vi "Standard Joystick Control.vi"() -> ()   [LabVIEW 2016, in "Aerotech VIs.lvlib"]
uses:
  Aerotech VIs.lvlib
  Motion/EnableMultiple.vi
  Motion/HomeSingle.vi
  Motion/MoveAbsMultiple.vi
  Motion/FaultAckMultiple.vi
  Motion/DisableMultiple.vi
panel:
  in  "PC Board Position":bool
  in  "Plate Position":bool
  in  "Silicon Position":bool
  out "Vacuum Working":bool[](array[boolean])
  in  "Vacuum On/Off":bool[](array[boolean])
  out "z vel units":string
  out "y vel units":string
  out "x vel units":string
  out "u vel units":string
  out "Z - Velocity":dbl
  out "Y - Velocity":dbl
  out "X - Velocity":dbl
  out "U - Velocity":dbl
  in  "Fault Acknowledged":bool
  in  "joystick reset":bool
  in  "joystick on":bool
  in  "stop":bool
  in  "z home":bool
  in  "y home":bool
  in  "x home":bool
  in  "u home":bool
  out "units 4":string
  out "units 3":string
  out "units 2":string
  out "units":string
  out "Z - Position":dbl
  out "Y - Position":dbl
  out "X - Position":dbl
  out "U - Position":dbl
  out "Z - Axis Status":string
  out "Y - Axis Status":string
  out "X - Axis Status":string
  out "U - Axis Status":string
  # "If vacuum sensor\nshows a green\nlight when turned\noffthen it means it\nis not wired correctly"
  # "Vacuum Controls"
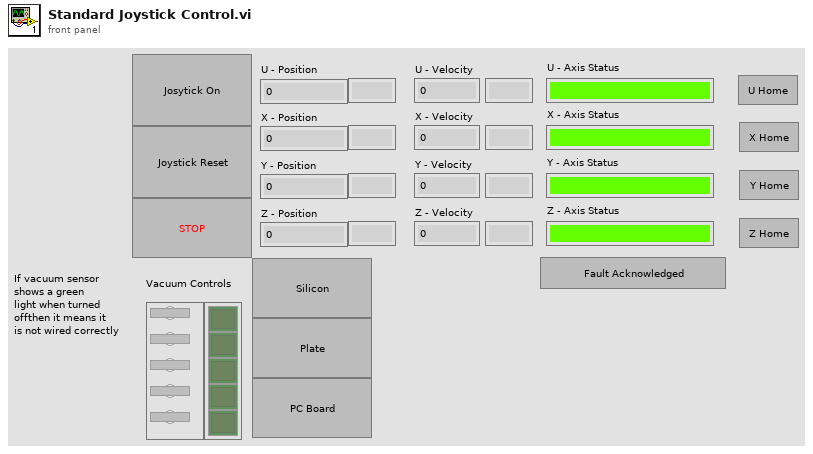
[diagram p1: front panel]
types:
  T1 = typedef "AxisDiagPacket.ctl" = cluster{"Axis Name":string, "Analog Input 0":dbl, "Analog Input 1":dbl, "Axis Fault (num)":i32, "Axis Fault (str)":string, "Axis Fault (bits)":cluster{"AmplifierFault":bool, "AmplifierTemperatureFault":bool, "CcwEndOfTravelLimitFault":bool, "CcwSoftwareLimitFault":bool, "CommunicationLostFault":bool, "CwEndOfTravelLimitFault":bool, "CwSoftwareLimitFault":bool, "EmergencyStopFault":bool, "EncoderFault":bool, "ExternalFault":bool, "FeedbackScalingFault":bool, "GantryMisalignFault ":bool, "HallSensorFault":bool, "InPositionTimeoutFault":bool, "MarkerSearchFault":bool, "MaxVelocityCommandFault":bool, "MotorTemperatureFault":bool, "None":bool, "OverCurrentFault":bool, "PositionErrorFault":bool, "PositionFeedbackFault":bool, "ProbeInputFault":bool, "SafeZoneFault":bool, "VelocityErrorFault":bool, "VelocityFeedbackFault":bool, "VoltageClampFault":bool, "PowerSupplyFault":bool}, "Axis Status (num)":i32, "Axis Status (str)":string, "Axis Status (bits)":cluster{"BacklashActive":bool, "CalibrationEnabled1D":bool, "CalibrationEnabled2D":bool, "CommandValid":bool, "DriveAbortPending":bool, "DrivePending":bool, "Enabling":bool, "GainMappingEnabled":bool, "GantryAligned":bool, "GantryRealigning":bool, "Homed":bool, "Homing":bool, "IFOVEnabled":bool, "Jogging":bool, "JogGenerating":bool, "JoystickControl":bool, "MasterSlaveControl":bool, "MotionBlocked":bool, "MotionClamped":bool, "MoveDone":bool, "None":bool, "NotVirtual":bool, "Profiling":bool, "Stability0":bool, "Stability1":bool, "TrajectoryFiltering":bool, "WaitDone":bool}, "Current Command":sgl, "Current Error":sgl, "Current Feedback":sgl, "Digital Inputs":i32, "Digital Outputs":i32, "Drive Status":i32, "Drive Status (str)":string, "Drive Status (bits)":cluster{"AccelerationPhase":bool, "AutofocusActive":bool, "BrakeOutput":bool, "CcwEndOfTravelLimitInput":bool, "CosineEncoderError":bool, "CurrentClamp":bool, "CwEndOfTravelLimitInput":bool, "DecelerationPhase":bool, "DualLoopActive":bool, "EmergencyStopInput":bool, "Enabled":bool, "EncoderClipping":bool, "GalvoCalibrationEnabled":bool, "GalvoPowerCorrection":bool, "HallAInput":bool, "HallBInput":bool, "HallCInput":bool, "HighResolutionMode":bool, "HomeLimitInput":bool, "InPosition":bool, "InPosition2":bool, "MarkerInput":bool, "MarkerLatch":bool, "MoveActive":bool, "NoMotorSupply":bool, "None":bool, "PowerLimiting":bool, "ProgrammingFlash":bool, "ProgrammingMXH":bool, "PSOHaltLatch":bool, "ServoControl":bool, "SineEncoderError":bool}, "Position Feedback Auxiliary":dbl, "Position Command":dbl, "Position Error":dbl, "Position Feedback":dbl, "Program Position Command":dbl, "Program Position Error":dbl, "Program Position Feedback":dbl, "Velocity Command":dbl, "Velocity Error":dbl, "Velocity Feedback":dbl}
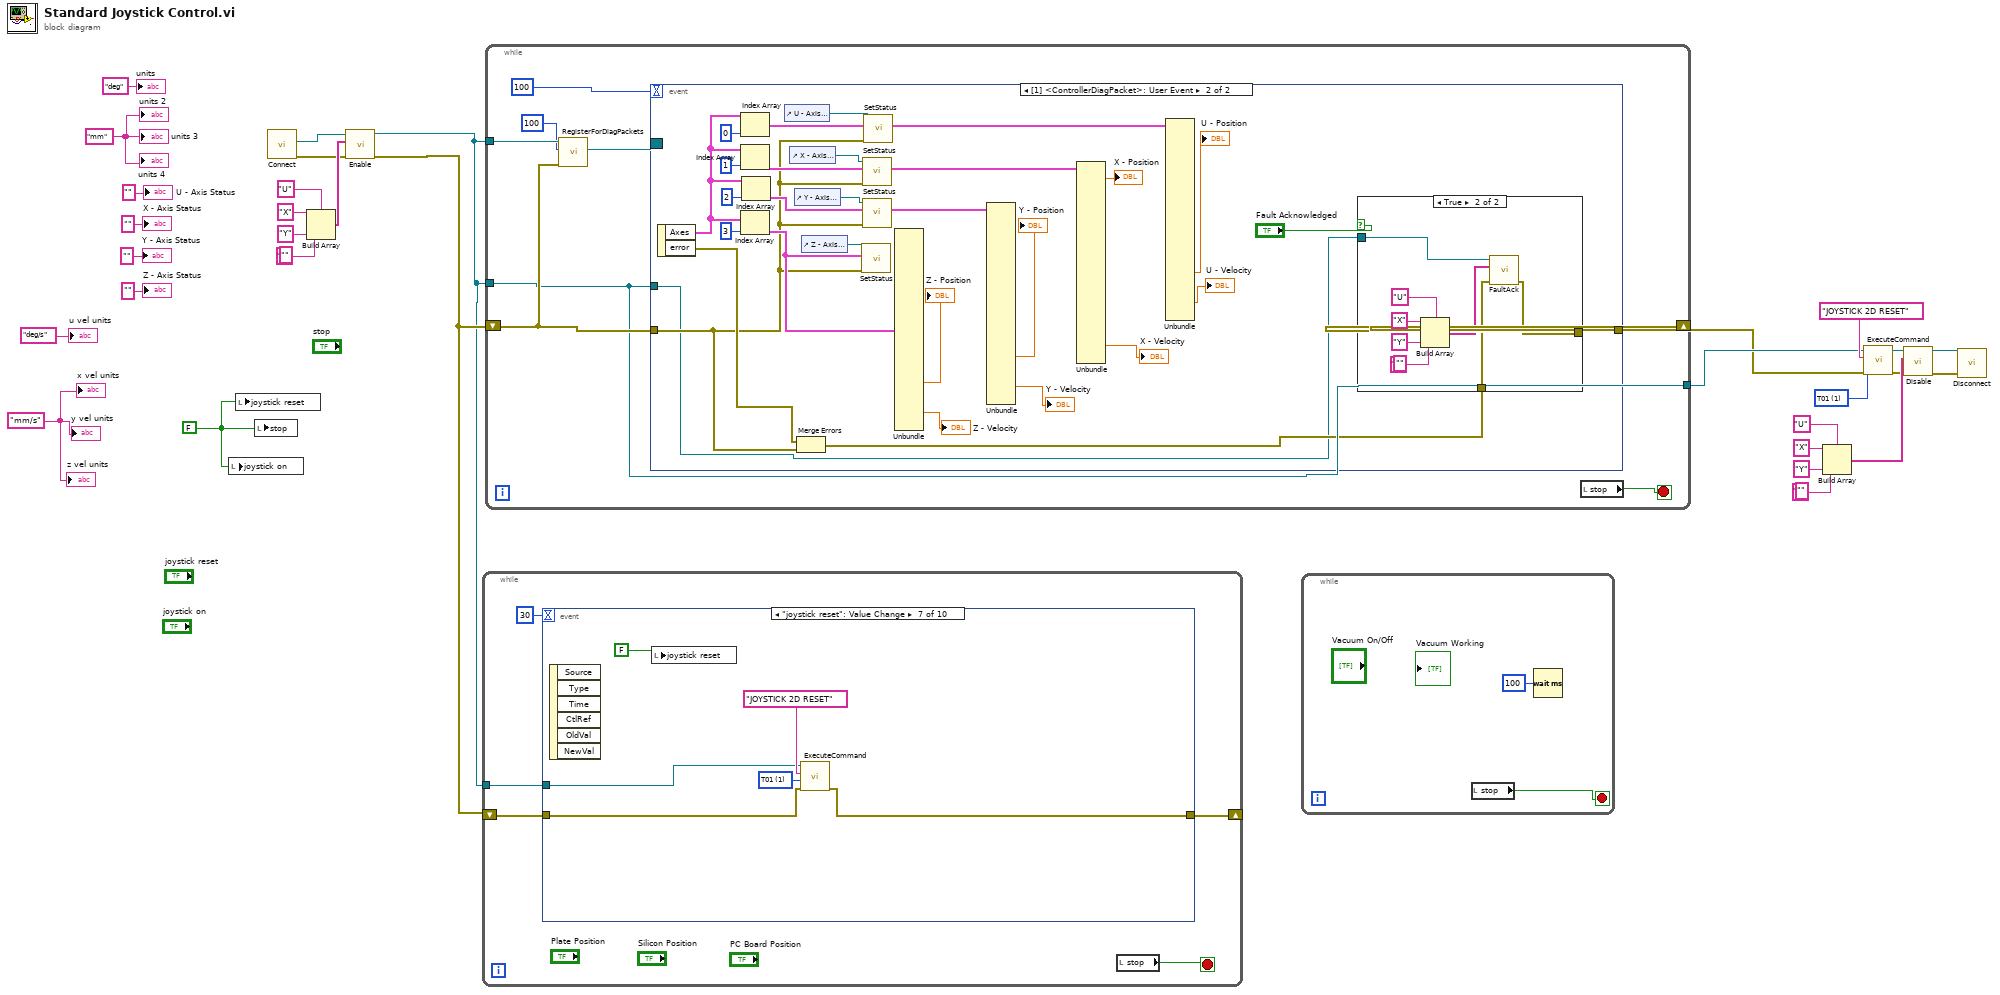
[diagram p0: block diagram]
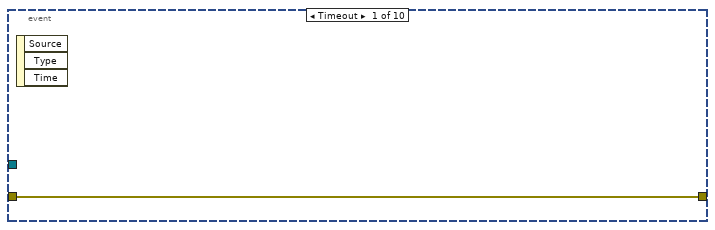
[diagram p2: hidden frame]
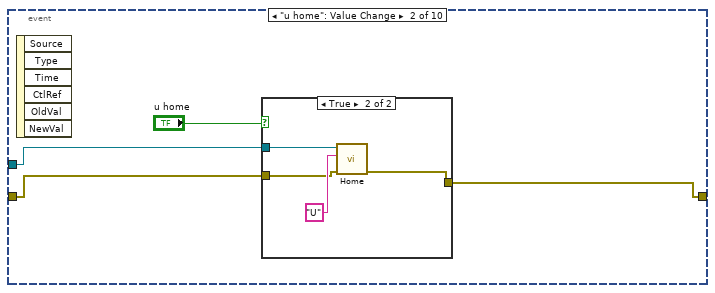
[diagram p3: hidden frame]
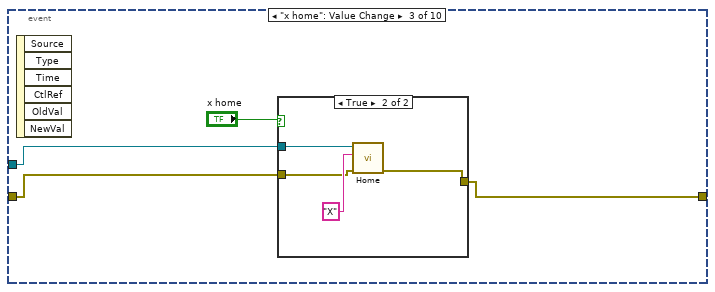
[diagram p5: hidden frame]
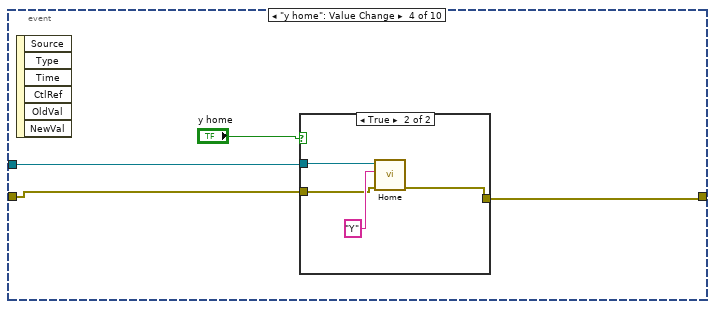
[diagram p7: hidden frame]
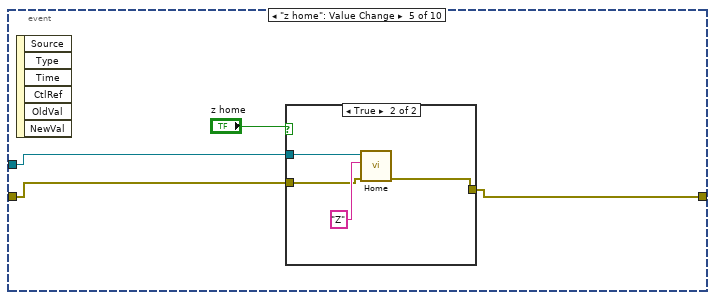
[diagram p9: hidden frame]
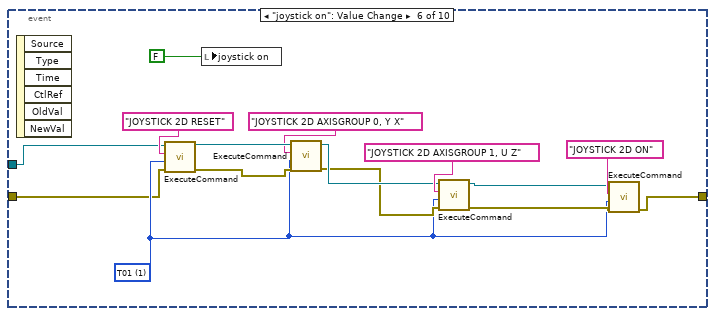
[diagram p11: hidden frame]
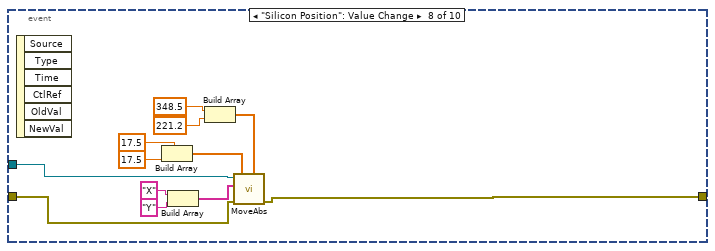
[diagram p12: hidden frame]
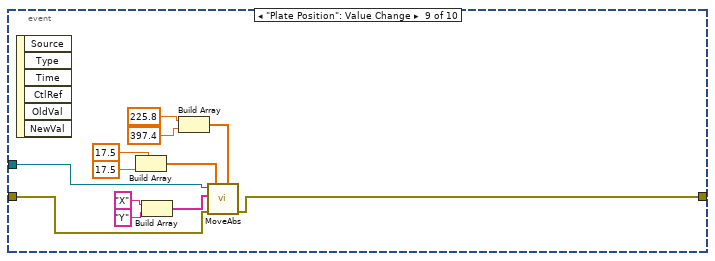
[diagram p13: hidden frame]
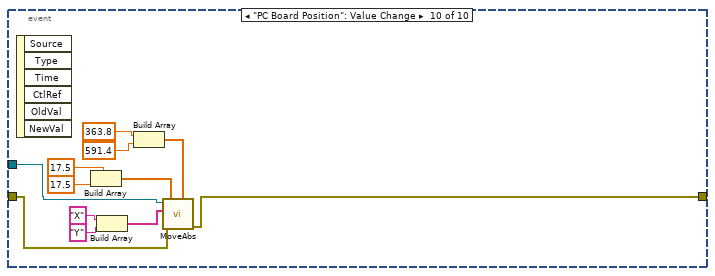
[diagram p14: hidden frame]
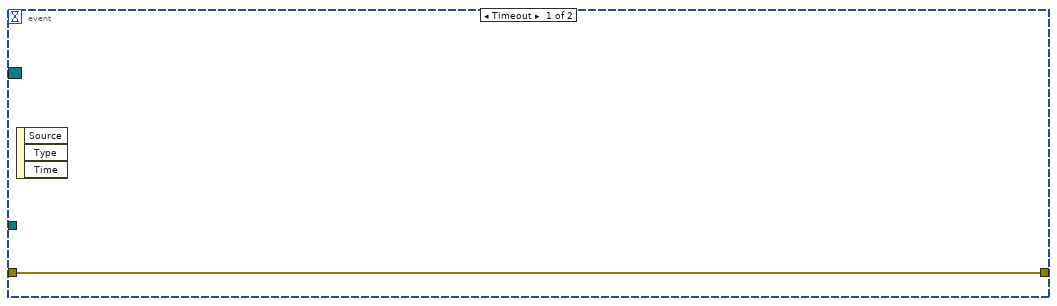
[diagram p15: hidden frame]
diagram:
  w9 = 1 items=["TLibrary", "T01", "T02", "T03", "T04", "T05", "T06", "T07", "T08", "T09", "T10", "T11", "T12", "T13", "T14", "T15", "T16", "T17", "T18", "T19", "T20", "T21", "T22", "T23", "T24", "T25", "T26", "T27", "T28", "T29", "T30", "T31"] ("taskId")
  w10 = "mm/s"
  w12 = FALSE
  (unwired) ""
  w19 = "mm"
  (unwired) ""
  n1 = local write "joystick on"(w12) -> ()
  n2 = local write "joystick reset"(w12) -> ()
  n3 = local write "stop"(w12) -> ()
  n4 = call "Connect.vi"() -> ("error out"=w22:errorcluster, "controller"=w21:refnum<k24>)  [unwired: 10 in]
  n5 = Build Array("U", "X", "Y", "Z") -> (w27:string[])
  n6 = call-poly "Enable.vi"("error in (no error)"=w22, "axis names"=w27, "controller in"=w21) -> ("error out"=w2:errorcluster, "controller out"=w1:refnum<k24>)  [unwired: 7 in]
  n7 = while {
    shift-right: [w35] -> _
    shift-left: w2 -> [w36]
    tunnel: w1 -> [w33]
    stop <- w32 stop-if-true
    n8 = event shown="[6] \"joystick reset\": Value Change" {
      selector: _ -> [_ _ _ _ _ _ _ _ _ _]
      dyn-events: _ -> [_ _ _ _ _ _ _ _ _ _]
      timeout: 30 -> [_ _ _ _ _ _ _ _ _ _]
      tunnel: w36 -> [w37 w41 w50 w59 w68 w75 w91 w105 w108 w120]
      tunnel: [w37 w40 w49 w58 w66 w74 w90 w104 w107 w119] -> w35
      tunnel: w33 -> [_ w39 w48 w57 w67 w76 w92 w106 w109 w121]
      event Timeout {
        n9 = event-data() -> ()  [unwired: 1 in, 3 out]
      }
      event "u home": Value Change {
        n10 = event-data() -> ()  [unwired: 1 in, 6 out]
        n11 = case shown="True" "u home" {
          tunnel: w41 -> [w42 w45]
          tunnel: [w42 w44] -> w40
          tunnel: w39 -> [_ w43]
          frame False {
          }
          frame True {
            n12 = call-poly "Home.vi"("error in (no error)"=w45, "axis name"="U", "controller in"=w43) -> ("error out"=w44:errorcluster)  [unwired: 7 in, 1 out]
          }
        }
      }
      event "x home": Value Change {
        n13 = event-data() -> ()  [unwired: 1 in, 6 out]
        n14 = case shown="True" "x home" {
          tunnel: w50 -> [w51 w54]
          tunnel: [w51 w53] -> w49
          tunnel: w48 -> [_ w52]
          frame False {
          }
          frame True {
            n15 = call-poly "Home.vi"("error in (no error)"=w54, "axis name"="X", "controller in"=w52) -> ("error out"=w53:errorcluster)  [unwired: 7 in, 1 out]
          }
        }
      }
      event "y home": Value Change {
        n16 = event-data() -> ()  [unwired: 1 in, 6 out]
        n17 = case shown="True" "y home" {
          tunnel: w59 -> [w60 w63]
          tunnel: [w60 w62] -> w58
          tunnel: w57 -> [_ w61]
          frame False {
          }
          frame True {
            n18 = call-poly "Home.vi"("error in (no error)"=w63, "axis name"="Y", "controller in"=w61) -> ("error out"=w62:errorcluster)  [unwired: 7 in, 1 out]
          }
        }
      }
      event "z home": Value Change {
        n19 = event-data() -> ()  [unwired: 1 in, 6 out]
        n20 = case shown="True" "z home" {
          tunnel: w68 -> [w69 w72]
          tunnel: [w69 w71] -> w66
          tunnel: w67 -> [_ w70]
          frame False {
          }
          frame True {
            n21 = call-poly "Home.vi"("error in (no error)"=w72, "axis name"="Z", "controller in"=w70) -> ("error out"=w71:errorcluster)  [unwired: 7 in, 1 out]
          }
        }
      }
      event "joystick on": Value Change {
        w77 = 1 items=["TLibrary", "T01", "T02", "T03", "T04", "T05", "T06", "T07", "T08", "T09", "T10", "T11", "T12", "T13", "T14", "T15", "T16", "T17", "T18", "T19", "T20", "T21", "T22", "T23", "T24", "T25", "T26", "T27", "T28", "T29", "T30", "T31"] ("taskId")
        n22 = event-data() -> ()  [unwired: 1 in, 6 out]
        n23 = call "ExecuteCommand.vi"("error in (no error)"=w75, "taskId"=w77, "Command Code"="JOYSTICK 2D RESET", "controller in"=w76) -> ("error out"=w86:errorcluster, "controller out"=w87:refnum<k24>)  [unwired: 5 in, 1 out]
        n24 = local write "joystick on"(FALSE) -> ()
        n25 = call "ExecuteCommand.vi"("error in (no error)"=w86, "taskId"=w77, "Command Code"="JOYSTICK 2D AXISGROUP 0, Y X", "controller in"=w87) -> ("error out"=w82:errorcluster, "controller out"=w83:refnum<k24>)  [unwired: 5 in, 1 out]
        n26 = call "ExecuteCommand.vi"("error in (no error)"=w82, "taskId"=w77, "Command Code"="JOYSTICK 2D AXISGROUP 1, U Z", "controller in"=w83) -> ("error out"=w80:errorcluster, "controller out"=w79:refnum<k24>)  [unwired: 5 in, 1 out]
        n27 = call "ExecuteCommand.vi"("error in (no error)"=w80, "taskId"=w77, "Command Code"="JOYSTICK 2D ON", "controller in"=w79) -> ("error out"=w74:errorcluster)  [unwired: 5 in, 2 out]
      }
      event "joystick reset": Value Change {
        w94 = 1 items=["TLibrary", "T01", "T02", "T03", "T04", "T05", "T06", "T07", "T08", "T09", "T10", "T11", "T12", "T13", "T14", "T15", "T16", "T17", "T18", "T19", "T20", "T21", "T22", "T23", "T24", "T25", "T26", "T27", "T28", "T29", "T30", "T31"] ("taskId")
        n28 = event-data() -> ()  [unwired: 1 in, 6 out]
        n29 = local write "joystick reset"(FALSE) -> ()
        n30 = call "ExecuteCommand.vi"("error in (no error)"=w91, "taskId"=w94, "Command Code"="JOYSTICK 2D RESET", "controller in"=w92) -> ("error out"=w90:errorcluster)  [unwired: 5 in, 2 out]
      }
      event "Silicon Position": Value Change {
        n31 = event-data() -> ()  [unwired: 1 in, 6 out]
        n32 = Build Array(17.5, 17.5) -> (w101:dbl[])
        n33 = Build Array("X", "Y") -> (w98:string[])
        n34 = Build Array(348.5, 221.2) -> (w95:dbl[])
        n35 = call-poly "MoveAbs.vi"("positions"=w95, "speeds"=w101, "error in (no error)"=w105, "axis names"=w98, "controller in"=w106) -> ("error out"=w104:errorcluster)  [unwired: 5 in, 1 out]
      }
      event "Plate Position": Value Change {
        n36 = event-data() -> ()  [unwired: 1 in, 6 out]
        n37 = Build Array(17.5, 17.5) -> (w116:dbl[])
        n38 = Build Array("X", "Y") -> (w113:string[])
        n39 = Build Array(225.8, 397.4) -> (w110:dbl[])
        n40 = call-poly "MoveAbs.vi"("positions"=w110, "speeds"=w116, "error in (no error)"=w108, "axis names"=w113, "controller in"=w109) -> ("error out"=w107:errorcluster)  [unwired: 5 in, 1 out]
      }
      event "PC Board Position": Value Change {
        n41 = event-data() -> ()  [unwired: 1 in, 6 out]
        n42 = Build Array(17.5, 17.5) -> (w128:dbl[])
        n43 = Build Array("X", "Y") -> (w125:string[])
        n44 = Build Array(363.8, 591.4) -> (w122:dbl[])
        n45 = call-poly "MoveAbs.vi"("positions"=w122, "speeds"=w128, "error in (no error)"=w120, "axis names"=w125, "controller in"=w121) -> ("error out"=w119:errorcluster)  [unwired: 5 in, 1 out]
      }
    }
    n46 = local read "stop"() -> (w32:bool)
  }
  n47 = while {
    tunnel: w1 -> [w132]
    shift-right: [w137] -> w3
    shift-left: w2 -> [w133]
    tunnel: w1 -> [w135]
    tunnel: [w132] -> w4
    stop <- w131 stop-if-true
    n48 = call "RegisterForDiagPackets.vi"("error in (no error)"=w133, "refresh interval (default)"=100, "Controller in"=w135) -> ("Event Registration Refnum"=w136:refnum<event-registration>)  [unwired: 4 in, 3 out]
    n49 = event shown="[1] <ControllerDiagPacket>: User Event" {
      selector: w136 -> [_ _]
      dyn-events: _ -> [_ _]
      timeout: 100 -> [_ _]
      tunnel: w133 -> [w139 w148]
      tunnel: w132 -> [_ w140]
      tunnel: [w139 w141] -> w137
      event Timeout {
        n50 = event-data() -> ()  [unwired: 1 in, 3 out]
      }
      event User Event {
        n51 = event-data() -> ("Axes"=w166:T1[], "error"=w149:errorcluster)  [unwired: 1 in]
        n52 = Index Array(array=w166, index=0) -> (element=w157:T1)
        n53 = Index Array(array=w166, index=1) -> (element=w155:T1)
        n54 = Index Array(array=w166, index=3) -> (element=w151:T1)
        n55 = Index Array(array=w166, index=2) -> (element=w153:T1)
        n56 = control-ref of="U - Axis Status"() -> (w161:refnum<vi>)
        n57 = control-ref of="X - Axis Status"() -> (w160:refnum<vi>)
        n58 = control-ref of="Y - Axis Status"() -> (w159:refnum<vi>)
        n59 = Merge Errors(w149, w148) -> (w142:errorcluster)
        n60 = control-ref of="Z - Axis Status"() -> (w158:refnum<vi>)
        n61 = call "SetStatus.vi"("error in (no error)"=w148, "AxisDiagPacket"=w151, "Status string"=w158) -> ()  [unwired: 8 in, 1 out]
        n62 = call "SetStatus.vi"("error in (no error)"=w148, "AxisDiagPacket"=w155, "Status string"=w160) -> ()  [unwired: 8 in, 1 out]
        n63 = call "SetStatus.vi"("error in (no error)"=w148, "AxisDiagPacket"=w153, "Status string"=w159) -> ()  [unwired: 8 in, 1 out]
        n64 = call "SetStatus.vi"("error in (no error)"=w148, "AxisDiagPacket"=w157, "Status string"=w161) -> ()  [unwired: 8 in, 1 out]
        n65 = Unbundle(w151) -> ("Position Feedback"=→"Z - Position":dbl, "Velocity Command"=→"Z - Velocity":dbl)  [unwired: 25 out]
        n66 = Unbundle(w153) -> ("Position Feedback"=→"Y - Position":dbl, "Velocity Command"=→"Y - Velocity":dbl)  [unwired: 25 out]
        n67 = Unbundle(w155) -> ("Position Feedback"=→"X - Position":dbl, "Velocity Command"=→"X - Velocity":dbl)  [unwired: 25 out]
        n68 = Unbundle(w157) -> ("Position Feedback"=→"U - Position":dbl, "Velocity Command"=→"U - Velocity":dbl)  [unwired: 25 out]
        n69 = case shown="True" "Fault Acknowledged" {
          tunnel: w142 -> [w167 w170]
          tunnel: [w167 w169] -> w141
          tunnel: w140 -> [_ w168]
          frame False {
          }
          frame True {
            (unwired) ""
            n70 = Build Array("U", "X", "Y", "Z") -> (w171:string[])
            n71 = call-poly "FaultAck.vi"("error in (no error)"=w170, "axis names"=w171, "controller in"=w168) -> ("error out"=w169:errorcluster)  [unwired: 7 in, 1 out]
          }
        }
      }
    }
    n72 = local read "stop"() -> (w131:bool)
  }
  n73 = while {
    stop <- w177 stop-if-true
    n74 = local read "stop"() -> (w177:bool)
    n75 = Wait (ms)(milliseconds to wait=u32 100) -> ()  [unwired: 1 out]
  }
  n76 = Build Array("U", "X", "Y", "Z") -> (w7:string[])
  n77 = call "ExecuteCommand.vi"("error in (no error)"=w3, "taskId"=w9, "Command Code"="JOYSTICK 2D RESET", "controller in"=w4) -> ("error out"=w6:errorcluster, "controller out"=w5:refnum<k24>)  [unwired: 5 in, 1 out]
  n78 = call-poly "Disable.vi"("error in (no error)"=w6, "axis names"=w7, "controller in"=w5) -> ("error out"=w14:errorcluster, "controller out"=w13:refnum<k24>)  [unwired: 7 in]
  n79 = call "Disconnect.vi"("error in (no error)"=w14, "controller"=w13) -> ()  [unwired: 9 in, 1 out]
  "U - Axis Status" <- "" ("U - Axis Status")
  "X - Axis Status" <- "" ("X - Axis Status")
  "Y - Axis Status" <- "" ("Y - Axis Status")
  "Z - Axis Status" <- "" ("Z - Axis Status")
  "units" <- "deg"
  "units 2" <- w19
  "units 3" <- w19
  "units 4" <- w19
  "u vel units" <- "deg/s"
  "x vel units" <- w10
  "y vel units" <- w10
  "z vel units" <- w10
